vi "Get_2N_Array_Length.vi"(1 "StringArray":string[][](array[string]), 2 "NumArray":i32[][](array[numeric])) -> (0 "Numeric":i32)   [LabVIEW 2014]
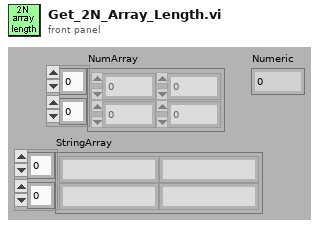
[diagram p1: front panel]
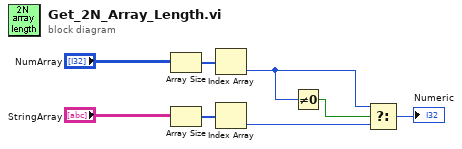
[diagram p0: block diagram]
diagram:
  n1 = Array Size(array="NumArray") -> (size(s)=w8:i32[])
  n2 = Array Size(array="StringArray") -> (size(s)=w6:i32[])
  n3 = Index Array(array=w8) -> (element=w3:i32)  [unwired: 1 in]
  n4 = Index Array(array=w6) -> (element=w2:i32)  [unwired: 1 in]
  n5 = Not Equal To 0?(x=w3) -> (x != 0?=w4:bool)
  n6 = Select(t=w3, s=w4, f=w2) -> (s? t:f=→"Numeric":i32)
